vi "test2.vi"() -> ()   [LabVIEW 2012]
uses:
  G_SEN.vi
panel:
  out "n0":i32
  out "errorsum":dbl[](array[numeric])
  out "seed0":bool[](array[boolean])
  out "y":dbl[](array[numeric])
  out "x":dbl[](array[numeric])
  out "Array 4":dbl[][](array[numeric])
  out "obs":dbl[][](array[numeric])
  out "x*y":dbl[](array[numeric])
  out "Array":dbl[][](array[numeric])
  out "XY Graph 2":cluster{"Y":dbl[], "Y":dbl[]}[](graph)
  out "Array 3":dbl[](array[numeric])
  out "Array 2":cluster{dbl[][]}[](array[cluster])
  out "error out":errorcluster
  out "XY Graph":cluster{"Y":dbl[], "Y":dbl[]}[](graph)
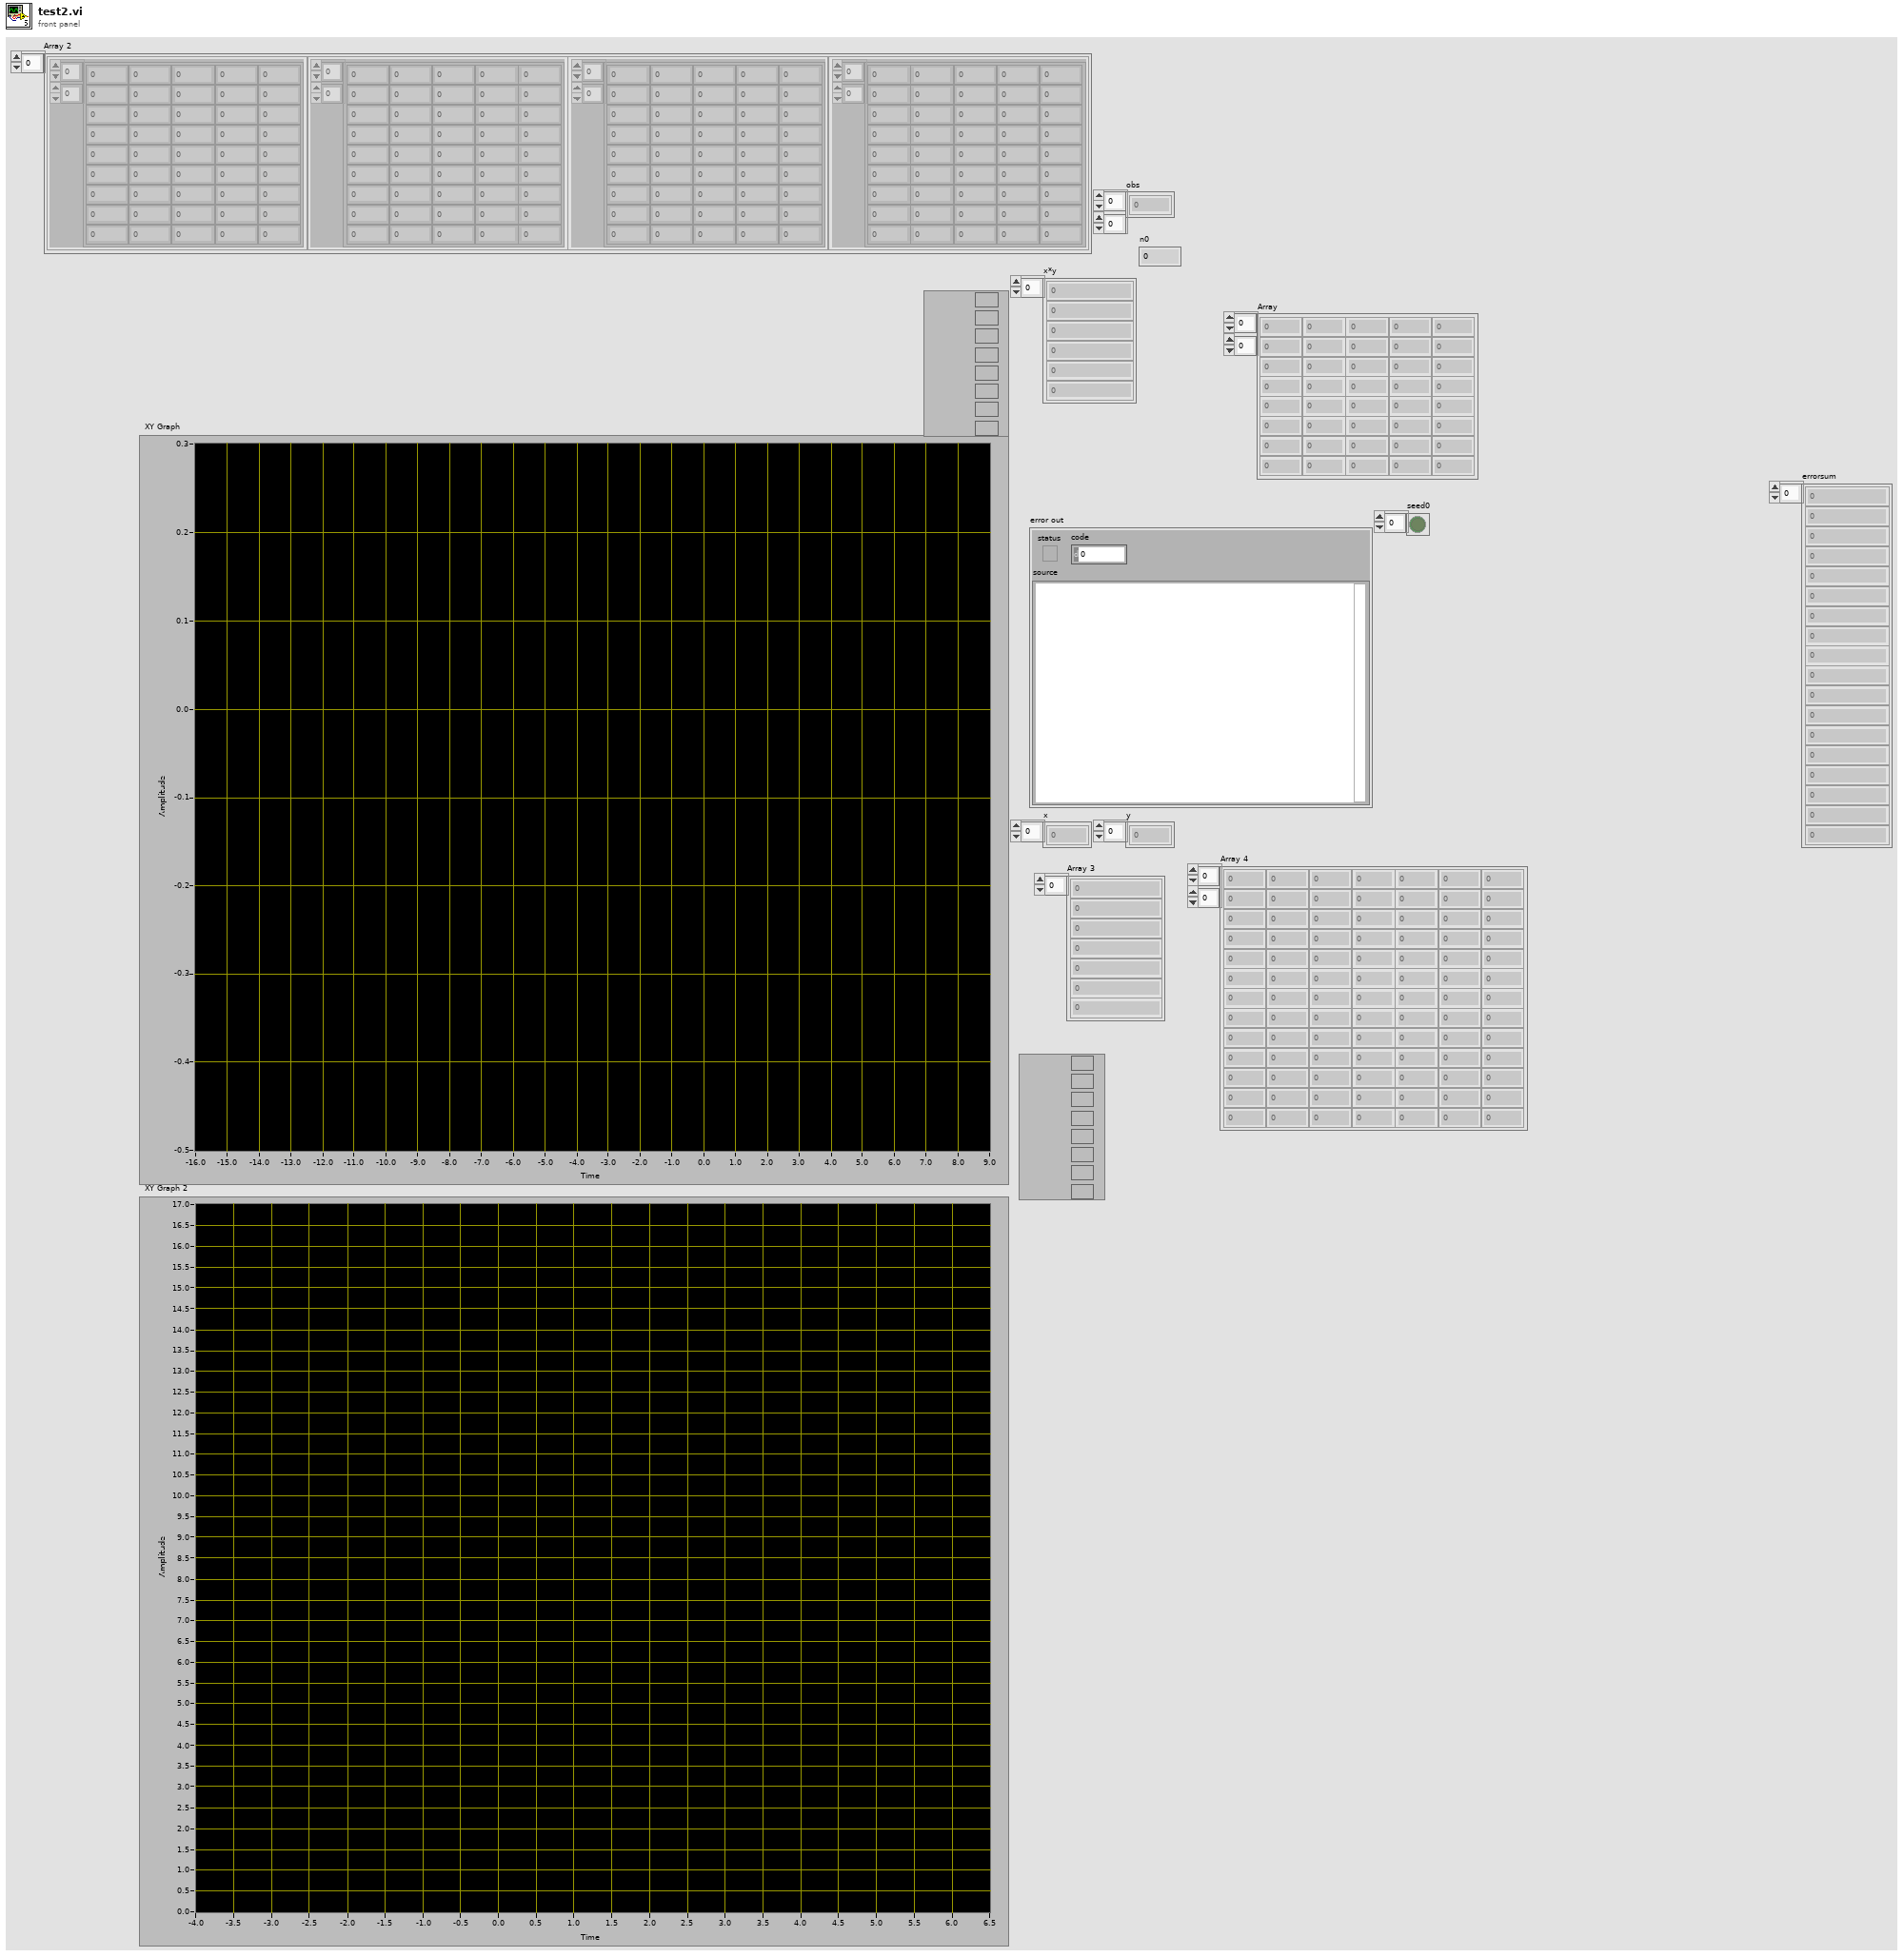
[diagram p1: front panel]
types:
  T1 = cluster{i16, "element":dbl, "element":dbl, "element":dbl, "element":dbl}[]
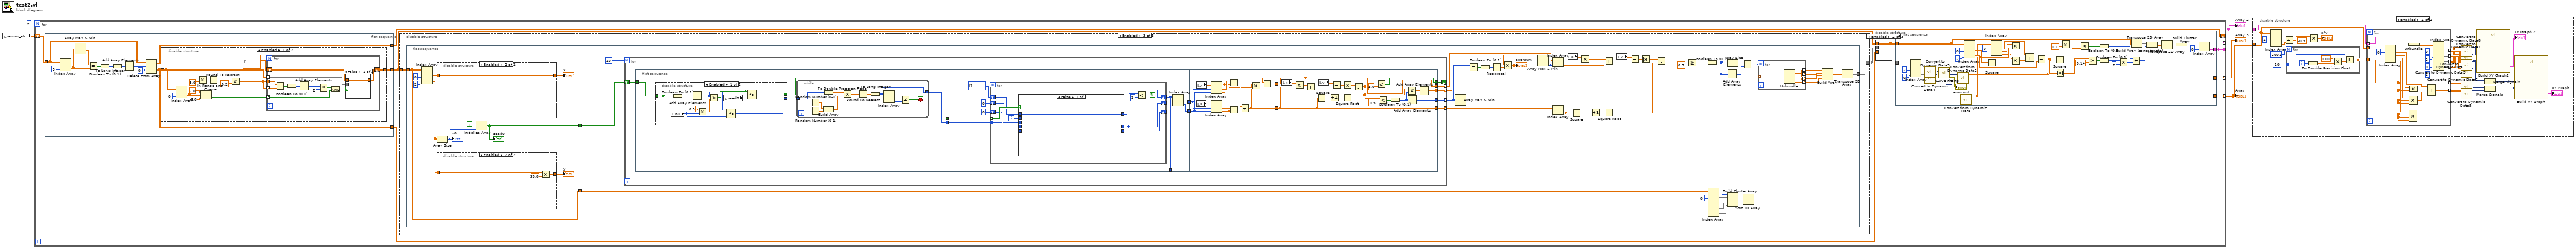
[diagram p0: block diagram]
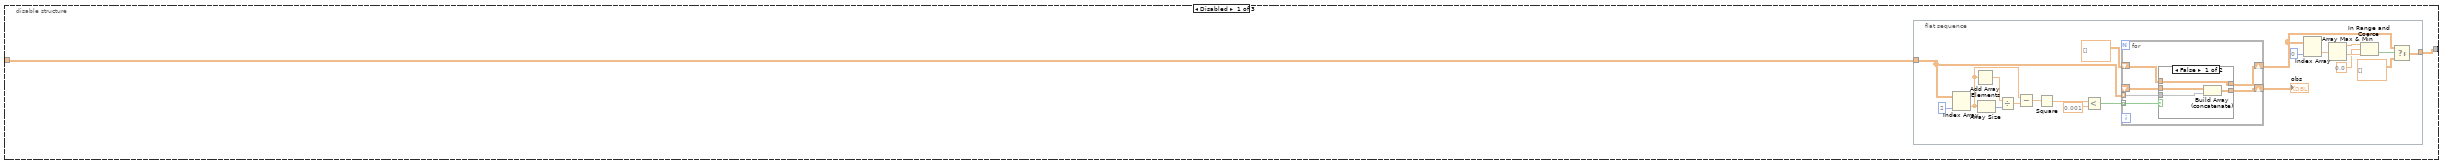
[diagram p3: hidden frame]
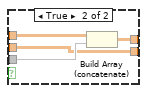
[diagram p4: hidden frame]
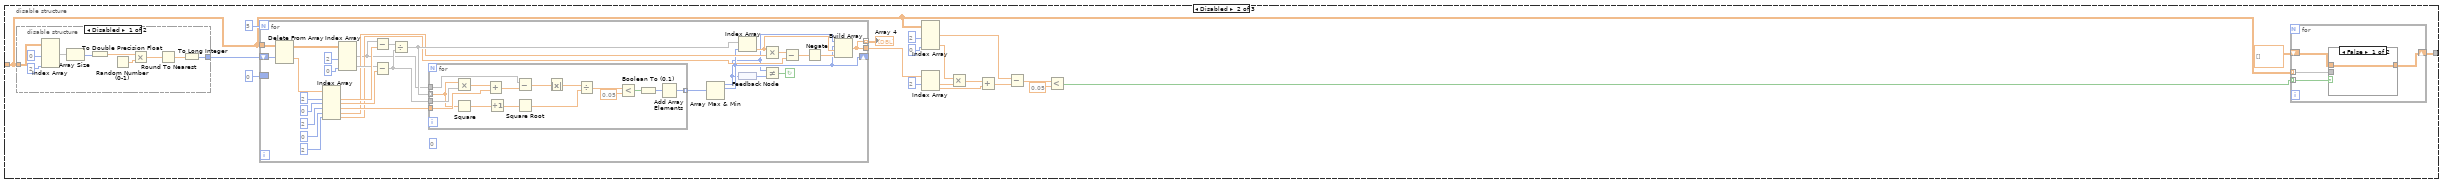
[diagram p5: hidden frame]
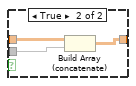
[diagram p6: hidden frame]
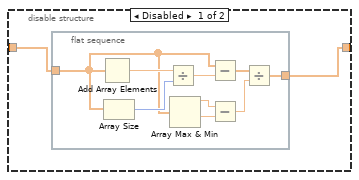
[diagram p8: hidden frame]
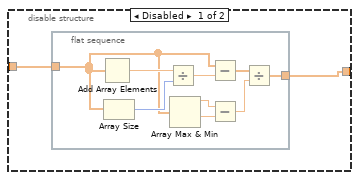
[diagram p9: hidden frame]
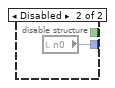
[diagram p10: hidden frame]
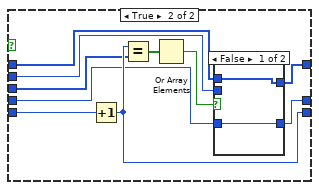
[diagram p11: hidden frame]
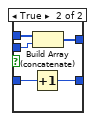
[diagram p12: hidden frame]
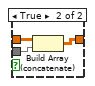
[diagram p13: hidden frame]
diagram:
  n1 = global read "G_SEN.vi" "sensor_etc"() -> (w4:dbl[][])
  n2 = for {
    N: 2 -> [_]
    shift-right: [w13] -> _
    shift-left: w4 -> [w14]
    tunnel: [w10] -> _
    tunnel: [w10] -> w2 mode=indexing
    tunnel: [w9] -> w3 mode=indexing
    tunnel: [w8] -> w1 mode=indexing
    n3 = flat-sequence {
      tunnel: w14 -> [w385]
      tunnel: [w382] -> w13
      tunnel: [w381] -> w12
      tunnel: [w380] -> w7
      frame #0 {
        n4 = Index Array(array=w385, index (col)=3 ("disabled index (col)")) -> (element=w389:dbl[])  [unwired: 1 in]
        n5 = Array Max & Min(array=w389) -> (min value=w390:dbl)  [unwired: 3 out]
        n6 = Equal?(x=w390, y=w389) -> (x = y?=w388:bool[])
        n7 = Boolean To (0,1)(Boolean=w388) -> (0, 1=w387:i16[])
        n8 = To Long Integer(number=w387) -> (32bit integer=w386:i32[])
        n9 = Add Array Elements(numeric array=w386) -> (sum=w384:i32)
        n10 = Delete From Array(array=w385, length=w384, index (row)=0) -> (deleted portion=w381:dbl[][], array with subset deleted=w382:dbl[][])  [unwired: 1 in]
        n11 = disable-structure shown="Enabled" {
          disable-tunnel: w381 -> [w397 w421]
          disable-tunnel: [w396 w421] -> w380
          frame Enabled {
            n12 = Index Array(array=w397, index (col)=0 ("disabled index (col)")) -> (element=w395:dbl[])  [unwired: 1 in]
            n13 = Multiply(x=w395, y=5.0) -> (x*y=w402:dbl[])
            n14 = In Range and Coerce(upper limit=7.0, x=w395, lower limit=-6.0) -> (In Range?=w393:bool[])  [unwired: 1 out]
            n15 = Round To Nearest(number=w402) -> (nearest integer value=w401:dbl[])
            n16 = Multiply(x=w401, y=0.2) -> (x*y=w399:dbl[])
            n17 = for {
              tunnel: w399 -> [w409] mode=indexing
              tunnel: w399 -> [w416]
              shift-right: [w412] -> w396
              shift-left: dbl[][] [] -> [w413]
              tunnel: w397 -> [w414] mode=indexing
              tunnel: w393 -> [w408] mode=indexing
              n18 = Equal?(x=w416, y=w409) -> (x = y?=w405:bool[])
              n19 = Boolean To (0,1)(Boolean=w405) -> (0, 1=w415:i16[])
              n20 = Add Array Elements(numeric array=w415) -> (sum=w411:i16)
              n21 = Less Or Equal?(x=w411, y=i16 2) -> (x <= y?=w407:bool)
              n22 = And(x=w407, y=w408) -> (x .and. y?=w406:bool)
              n23 = case shown="False" w406 {
                tunnel: w414 -> [_ w420]
                tunnel: w413 -> [w417 w419]
                tunnel: [w417 w418] -> w412
                frame False {
                }
                frame True {
                  n24 = Build Array (concatenate)(w419, w420) -> (w418:dbl[][])
                }
              }
            }
          }
          frame Disabled {
          }
        }
      }
    }
    n25 = disable-structure shown="Enabled" {
      disable-tunnel: [w16 w54 w137] -> w11
      disable-tunnel: w7 -> [w15 w56 w138]
      frame Disabled {
        n26 = flat-sequence {
          tunnel: [w37] -> w16
          tunnel: w15 -> [w36]
          frame #0 {
            n27 = Index Array(array=w36, index (col)=2 ("disabled index (col)")) -> (element=w23:dbl[])  [unwired: 1 in]
            n28 = Add Array Elements(numeric array=w23) -> (sum=w26:dbl)
            n29 = Array Size(array=w23) -> (size(s)=w22:i32)
            n30 = Divide(x=w26, y=w22) -> (x/y=w25:dbl)
            n31 = Subtract(x=w23, y=w25) -> (x-y=w24:dbl[])
            n32 = Square(x=w24) -> (x^2=w21:dbl[])
            n33 = Less?(x=w21, y=0.001) -> (x < y?=w19:bool[])
            n34 = for {
              tunnel: w36 -> [w42] mode=indexing
              tunnel: w19 -> [w43] mode=indexing
              shift-right: [w40] -> w29
              shift-left: dbl[][] [] -> [w41]
              shift-right: [w38] -> w17
              shift-left: _ -> [w39]
              n35 = case shown="False" w43 {
                tunnel: w42 -> [w46 w51]
                tunnel: w41 -> [w47 w50]
                tunnel: [w47 w49] -> w40
                tunnel: w39 -> [w45 w48]
                tunnel: [w44 w48] -> w38
                frame False {
                  n36 = Build Array (concatenate)(w45, w46) -> (w44:dbl[][])
                }
                frame True {
                  n37 = Build Array (concatenate)(w50, w51) -> (w49:dbl[][])
                }
              }
            }
            "obs" <- w17
            n38 = Index Array(array=w29, index (col)=0 ("disabled index (col)")) -> (element=w34:dbl[])  [unwired: 1 in]
            n39 = Array Max & Min(array=w34) -> (max value=w33:dbl, min value=w32:dbl)  [unwired: 2 out]
            n40 = In Range and Coerce(upper limit=w33, x=0.0, lower limit=w32) -> (In Range?=w30:bool)  [unwired: 1 out]
            n41 = Select(t=w29, s=w30, f=dbl[][] []) -> (s? t:f=w37:dbl[][])
          }
        }
      }
      frame Disabled {
        n42 = disable-structure shown="Disabled" {
          disable-tunnel: w56 -> [w85 _]
          disable-tunnel: [w80 _] -> w71
          frame Disabled {
            n43 = Index Array(array=w85, index (col) #1=0 ("disabled index (col)"), index (col) #2=2 ("index (col)")) -> (element #1=w87:dbl[])  [unwired: 2 in, 1 out]
            n44 = Array Size(array=w87) -> (size(s)=w86:i32)
            n45 = To Double Precision Float(number=w86) -> (double precision float=w84:dbl)
            n46 = Random Number (0-1)() -> (number: 0 to 1=w83:dbl)
            n47 = Multiply(x=w84, y=w83) -> (x*y=w82:dbl)
            n48 = Round To Nearest(number=w82) -> (nearest integer value=w81:dbl)
            n49 = To Long Integer(number=w81) -> (32bit integer=w80:i32)
          }
          frame Enabled {
          }
        }
        n50 = for {
          N: 5 -> [_]
          tunnel: w56 -> [w120]
          tunnel: [w90] -> w67
          shift-right: [w94] -> _
          shift-left: w71 -> [w119]
          tunnel: [w90] -> w53 mode=indexing
          border: i16 0 -> [_]
          stop <- w91 continue-if-true
          (unwired) i16 0
          n51 = Delete From Array(array=w120, index (row)=w119) -> (deleted portion=w115:dbl[], array with subset deleted=w118:dbl[][])  [unwired: 2 in]
          n52 = Index Array(array=w115, index #1=2 ("disabled index (col)"), index #2=0 ("index (col)"), index #3=2 ("index"), index #4=0 ("index"), index #5=2 ("index")) -> (element #1=w112:dbl, element #2=w110:dbl, element #3=w106:dbl, element #4=w102:dbl, element #5=w99:dbl)
          n53 = Index Array(array=w118, index (col) #1=2 ("disabled index (col)"), index (col) #2=0 ("index (col)")) -> (element #1=w95:dbl[], element #2=w111:dbl[])  [unwired: 2 in]
          n54 = Subtract(x=w95, y=w112) -> (x-y=w109:dbl[])
          n55 = Subtract(x=w111, y=w110) -> (x-y=w108:dbl[])
          n56 = Divide(x=w109, y=w108) -> (x/y=w104:dbl[])
          n57 = for {
            tunnel: w104 -> [w128] mode=indexing
            tunnel: w108 -> [w136]
            tunnel: w106 -> [w134]
            tunnel: w95 -> [w132]
            tunnel: [w121] -> w105 mode=indexing
            n58 = Multiply(x=w128, y=w136) -> (x*y=w135:dbl[])
            n59 = Square(x=w128) -> (x^2=w127:dbl)
            n60 = Add(x=w135, y=w134) -> (x+y=w133:dbl[])
            n61 = Increment(x=w127) -> (x+1=w126:dbl)
            n62 = Subtract(x=w132, y=w133) -> (x-y=w131:dbl[])
            n63 = Square Root(x=w126) -> (sqrt(x)=w125:dbl)
            n64 = Absolute Value(x=w131) -> (abs(x)=w124:dbl[])
            n65 = Divide(x=w124, y=w125) -> (x/y=w123:dbl[])
            n66 = Less?(x=w123, y=0.05) -> (x < y?=w129:bool[])
            n67 = Boolean To (0,1)(Boolean=w129) -> (0, 1=w122:i16[])
            n68 = Add Array Elements(numeric array=w122) -> (sum=w121:i16)
          }
          n69 = Array Max & Min(array=w105) -> (max value=w92:i16, max index (indices)=w94:i32)  [unwired: 2 out]
          n70 = Index Array(array=w104, index=w94) -> (element=w96:dbl)
          n71 = feedback-in #1(w92) -> ()
          n72 = feedback #1() -> (w93:i16)
          n73 = Multiply(x=w96, y=w102) -> (x*y=w101:dbl)
          n74 = Not Equal?(x=w92, y=w93) -> (x != y?=w91:bool)
          n75 = Subtract(x=w101, y=w99) -> (x-y=w98:dbl)
          n76 = Negate(x=w98) -> (-x=w97:dbl)
          n77 = Build Array(w92, w94, w96, w97) -> (w90:dbl[])
        }
        "Array 4" <- w53
        n78 = Index Array(array=w56, index (col) #1=2 ("disabled index (col)"), index (col) #2=0 ("index (col)")) -> (element #1=w60:dbl[], element #2=w64:dbl[])  [unwired: 2 in]
        n79 = Index Array(array=w67, index #1=2 ("index")) -> (element #1=w65:dbl, element #2=w62:dbl)  [unwired: 1 in]
        n80 = Multiply(x=w64, y=w65) -> (x*y=w63:dbl[])
        n81 = Add(x=w63, y=w62) -> (x+y=w61:dbl[])
        n82 = Subtract(x=w60, y=w61) -> (x-y=w58:dbl[])
        n83 = Less?(x=w58, y=0.05) -> (x < y?=w57:bool[])
        n84 = for {
          tunnel: w57 -> [w75] mode=indexing
          tunnel: w56 -> [w74] mode=indexing
          shift-right: [w73] -> w54
          shift-left: dbl[][] [] -> [w72]
          n85 = case shown="False" w75 {
            tunnel: w74 -> [_ w79]
            tunnel: [w76 w78] -> w73
            tunnel: w72 -> [w76 w77]
            frame False {
            }
            frame True {
              n86 = Build Array (concatenate)(w77, w79) -> (w78:dbl[][])
            }
          }
        }
      }
      frame Enabled {
        n87 = flat-sequence {
          tunnel: w138 -> [w145]
          tunnel: [w146] -> w140
          tunnel: [w145] -> w139
          tunnel: w140 -> [w220]
          tunnel: w139 -> [w205]
          tunnel: [w194] -> w137
          frame #0 {
            n88 = Index Array(array=w145, index (col) #1=0 ("disabled index (col)"), index (col) #2=2 ("index (col)")) -> (element #1=w144:dbl[], element #2=w142:dbl[])  [unwired: 2 in]
            n89 = disable-structure shown="Enabled" {
              disable-tunnel: w144 -> [w152 w162]
              disable-tunnel: [w151 w162] -> w143
              frame Disabled {
                n90 = flat-sequence {
                  tunnel: w152 -> [w156]
                  tunnel: [w153] -> w151
                  frame #0 {
                    n91 = Add Array Elements(numeric array=w156) -> (sum=w159:dbl)
                    n92 = Array Size(array=w156) -> (size(s)=w158:i32)
                    n93 = Divide(x=w159, y=w158) -> (x/y=w157:dbl)
                    n94 = Array Max & Min(array=w156) -> (max value=w161:dbl, min value=w160:dbl)  [unwired: 2 out]
                    n95 = Subtract(x=w156, y=w157) -> (x-y=w155:dbl[])
                    n96 = Subtract(x=w161, y=w160) -> (x-y=w154:dbl)
                    n97 = Divide(x=w155, y=w154) -> (x/y=w153:dbl[])
                  }
                }
              }
              frame Enabled {
              }
            }
            "x" <- w143
            n98 = Array Size(array=w142) -> (size(s)=w148:i32)
            "n0" <- w148
            n99 = disable-structure shown="Enabled" {
              disable-tunnel: w142 -> [w164 w176]
              disable-tunnel: [w163 w175] -> w141
              frame Disabled {
                n100 = flat-sequence {
                  tunnel: w164 -> [w168]
                  tunnel: [w165] -> w163
                  frame #0 {
                    n101 = Add Array Elements(numeric array=w168) -> (sum=w171:dbl)
                    n102 = Array Size(array=w168) -> (size(s)=w170:i32)
                    n103 = Divide(x=w171, y=w170) -> (x/y=w169:dbl)
                    n104 = Array Max & Min(array=w168) -> (max value=w173:dbl, min value=w172:dbl)  [unwired: 2 out]
                    n105 = Subtract(x=w168, y=w169) -> (x-y=w167:dbl[])
                    n106 = Subtract(x=w173, y=w172) -> (x-y=w166:dbl)
                    n107 = Divide(x=w167, y=w166) -> (x/y=w165:dbl[])
                  }
                }
              }
              frame Enabled {
                n108 = Multiply(x=w176, y=30.0) -> (x*y=w175:dbl[])
              }
            }
            "y" <- w141
            n109 = Initialize Array(TRUE, w148) -> (w146:bool[])
            "seed0" <- w146
          }
          frame #1 {
            n110 = for {
              N: 20 -> [_]
              shift-right: [w232] -> _
              shift-left: w220 -> [w235]
              tunnel: [w231] -> w218 mode=indexing
              tunnel: [w230] -> w217 mode=indexing
              tunnel: [w227] -> w184 mode=indexing
              tunnel: [w226] -> w188 mode=indexing
              n111 = flat-sequence {
                tunnel: w235 -> [w241]
                tunnel: [w238] -> w234
                tunnel: [w240] -> w233
                tunnel: [w266] -> w237
                tunnel: [w265] -> w236
                tunnel: w234 -> [w271]
                tunnel: w233 -> [w269]
                tunnel: [w264] -> _
                tunnel: w237 -> [w313]
                tunnel: w236 -> [w312]
                tunnel: [w304] -> w229
                tunnel: [w303] -> w228
                tunnel: [w330] -> w232
                tunnel: [w321] -> w231
                tunnel: [w329] -> w230
                tunnel: w229 -> [w329]
                tunnel: w228 -> [w321]
                tunnel: [w325] -> w227
                tunnel: [w324] -> w226
                frame #0 {
                  n112 = disable-structure shown="Enabled" {
                    disable-tunnel: w241 -> [w245 _]
                    disable-tunnel: [w247 w252] -> w239
                    disable-tunnel: [w244 _] -> w238
                    frame Enabled {
                      n113 = local read "n0"() -> (w246:i32)
                      n114 = Boolean To (0,1)(Boolean=w245) -> (0, 1=w251:i16[])
                      n115 = Add Array Elements(numeric array=w251) -> (sum=w248:i16)
                      n116 = Multiply(x=0.5, y=w246) -> (x*y=w249:dbl)
                      n117 = Greater?(x=w248, y=w249) -> (0:w242:bool)
                      n118 = local read "seed0"() -> (w243:bool[])
                      n119 = Select(t=w248, s=w242, f=w246) -> (s? t:f=w247:i32)
                      n120 = Select(t=w245, s=w242, f=w243) -> (s? t:f=w244:bool[])
                    }
                    frame Disabled {
                      n121 = local read "n0"() -> (w252:i32)
                    }
                  }
                  n122 = while {
                    tunnel: w239 -> [w254]
                    tunnel: [w253] -> w240
                    stop <- w255 stop-if-true
                    n123 = Random Number (0-1)() -> (number: 0 to 1=w263:dbl)
                    n124 = Random Number (0-1)() -> (number: 0 to 1=w262:dbl)
                    n125 = Build Array(w263, w262) -> (w261:dbl[])
                    n126 = To Double Precision Float(number=w254) -> (double precision float=w258:dbl)
                    n127 = Multiply(x=w258, y=w261) -> (x*y=w260:dbl[])
                    n128 = Round To Nearest(number=w260) -> (nearest integer value=w259:dbl[])
                    n129 = To Long Integer(number=w259) -> (32bit integer=w253:i32[])
                    n130 = Index Array(array=w253) -> (element #1=w257:i32, element #2=w256:i32)  [unwired: 2 in]
                    n131 = Not Equal?(x=w257, y=w256) -> (x != y?=w255:bool)
                  }
                }
                frame #1 {
                  n132 = for {
                    tunnel: w271 -> [w282] mode=indexing
                    shift-right: [w280] -> _
                    shift-left: 0 -> [w281]
                    tunnel: w269 -> [w279]
                    shift-right: [w277] -> w264
                    shift-left: i32[] [] -> [w276]
                    shift-right: [w274] -> _
                    shift-left: 0 -> [w275]
                    i -> [w278]
                    stop <- w272 continue-if-true
                    n133 = case shown="False" w282 {
                      tunnel: w281 -> [w285 w295]
                      tunnel: [w285 w294] -> w280
                      tunnel: w279 -> [_ w293]
                      tunnel: w278 -> [_ w290]
                      tunnel: [w284 w289] -> w277
                      tunnel: w276 -> [w284 w288]
                      tunnel: w275 -> [w283 w287]
                      tunnel: [w283 w286] -> w274
                      frame False {
                      }
                      frame True {
                        n134 = Increment(x=w295) -> (x+1=w294:i32)
                        n135 = Equal?(x=w294, y=w293) -> (x = y?=w292:bool[])
                        n136 = Or Array Elements(Boolean array=w292) -> (logical OR=w291:bool)
                        n137 = case shown="False" w291 {
                          tunnel: w290 -> [_ w302]
                          tunnel: [w297 w301] -> w289
                          tunnel: w288 -> [w297 w300]
                          tunnel: w287 -> [w296 w299]
                          tunnel: [w296 w298] -> w286
                          frame False {
                          }
                          frame True {
                            n138 = Increment(x=w299) -> (x+1=w298:i32)
                            n139 = Build Array (concatenate)(w300, w302) -> (w301:i32[])
                          }
                        }
                      }
                    }
                    n140 = Less?(x=w274, y=2) -> (x < y?=w272:bool)
                  }
                  n141 = Index Array(array=w264) -> (element #1=w266:i32, element #2=w265:i32)  [unwired: 2 in]
                }
                frame #2 {
                  n142 = local read "y"() -> (w314:dbl[])
                  n143 = local read "x"() -> (w315:dbl[])
                  n144 = Index Array(array=w315, index #1=w313, index #2=w312) -> (element #1=w309:dbl, element #2=w306:dbl)
                  n145 = Index Array(array=w314, index #1=w313, index #2=w312) -> (element #1=w307:dbl, element #2=w305:dbl)
                  n146 = Subtract(x=w307, y=w305) -> (x-y=w311:dbl)
                  n147 = Subtract(x=w309, y=w306) -> (x-y=w310:dbl)
                  n148 = Divide(x=w311, y=w310) -> (x/y=w303:dbl)
                  n149 = Multiply(x=w303, y=w306) -> (x*y=w308:dbl)
                  n150 = Subtract(x=w305, y=w308) -> (x-y=w304:dbl)
                }
                frame #3 {
                  n151 = local read "x"() -> (w328:dbl[])
                  n152 = Multiply(x=w328, y=w321) -> (x*y=w335:dbl[])
                  n153 = Add(x=w335, y=w329) -> (x+y=w334:dbl[])
                  n154 = Square(x=w321) -> (x^2=w320:dbl)
                  n155 = local read "y"() -> (w333:dbl[])
                  n156 = Increment(x=w320) -> (x+1=w319:dbl)
                  n157 = Subtract(x=w333, y=w334) -> (x-y=w332:dbl[])
                  n158 = Absolute Value(x=w332) -> (abs(x)=w318:dbl[])
                  n159 = Square Root(x=w319) -> (sqrt(x)=w317:dbl)
                  n160 = Divide(x=w318, y=w317) -> (x/y=w316:dbl[])
                  n161 = Less?(x=w316, y=3.0) -> (x < y?=w330:bool[])
                  n162 = Less?(x=w316, y=0.5) -> (x < y?=w322:bool[])
                  n163 = Boolean To (0,1)(Boolean=w322) -> (0, 1=w326:i16[])
                  n164 = Multiply(x=w316, y=w326) -> (x*y=w327:dbl[])
                  n165 = Add Array Elements(numeric array=w326) -> (sum=w324:i16)
                  n166 = Add Array Elements(numeric array=w327) -> (sum=w325:dbl)
                }
              }
            }
            n167 = Array Max & Min(array=w188) -> (max value=w189:i16)  [unwired: 3 out]
            n168 = Equal?(x=w188, y=w189) -> (x = y?=w187:bool[])
            n169 = Boolean To (0,1)(Boolean=w187) -> (0, 1=w186:i16[])
            n170 = Reciprocal(x=w186) -> (1/x=w185:dbl[])
            n171 = Multiply(x=w184, y=w185) -> (x*y=w183:dbl[])
            "errorsum" <- w183
            n172 = Array Max & Min(array=w183) -> (min index (indices)=w216:i32)  [unwired: 3 out]
            n173 = Index Array(array=w217, index=w216) -> (element=w209:dbl)
            n174 = Index Array(array=w218, index=w216) -> (element=w179:dbl)
            n175 = local read "x"() -> (w215:dbl[])
            n176 = Square(x=w179) -> (x^2=w180:dbl)
            n177 = Multiply(x=w215, y=w179) -> (x*y=w210:dbl[])
            n178 = Increment(x=w180) -> (x+1=w181:dbl)
            n179 = Add(x=w210, y=w209) -> (x+y=w211:dbl[])
            n180 = Square Root(x=w181) -> (sqrt(x)=w182:dbl)
            n181 = local read "y"() -> (w212:dbl[])
            n182 = Subtract(x=w212, y=w211) -> (x-y=w213:dbl[])
            n183 = Absolute Value(x=w213) -> (abs(x)=w178:dbl[])
            n184 = Divide(x=w178, y=w182) -> (x/y=w177:dbl[])
            n185 = Greater Or Equal?(x=w177, y=0.5) -> (x >= y?=w208:bool[])
            n186 = Boolean To (0,1)(Boolean=w208) -> (0, 1=w193:i16[])
            n187 = Index Array(array=w205, index (col) #1=0 ("disabled index (col)")) -> (element #1=w203:dbl[], element #2=w202:dbl[], element #3=w201:dbl[], element #4=w200:dbl[])  [unwired: 7 in]
            n188 = Add Array Elements(numeric array=w193) -> (sum=w191:i16)
            n189 = Array Size(array=w193) -> (size(s)=w192:i32)
            n190 = Build Cluster Array(w193, w203, w202, w201, w200) -> (w207:T1)
            n191 = Subtract(x=w192, y=w191) -> (x-y=w190:i32)
            n192 = Sort 1D Array(array=w207) -> (sorted array=w206:T1)
            n193 = for {
              N: w190 -> [_]
              tunnel: w206 -> [w225] mode=indexing
              tunnel: [w224] -> w199 mode=indexing
              tunnel: [w223] -> w198 mode=indexing
              tunnel: [w222] -> w197 mode=indexing
              tunnel: [w221] -> w196 mode=indexing
              n194 = Unbundle(w225) -> ("element"=w224:dbl, "element"=w223:dbl, "element"=w222:dbl, "element"=w221:dbl)  [unwired: 1 out]
            }
            n195 = Build Array(w199, w198, w197, w196) -> (w195:dbl[][])
            n196 = Transpose 2D Array(2D array=w195) -> (transposed array=w194:dbl[][])
          }
        }
      }
    }
    n197 = disable-structure shown="Enabled" {
      disable-tunnel: w12 -> [w422 _ _]
      disable-tunnel: [w422 w423 w424] -> w6
      disable-tunnel: w11 -> [_ _ w424]
      disable-tunnel: w7 -> [_ w423 _]
      frame Disabled {
      }
      frame Enabled {
      }
      frame Disabled {
      }
    }
    n198 = flat-sequence {
      tunnel: w11 -> [w340]
      tunnel: [w339] -> w10
      tunnel: [w338] -> w9
      tunnel: [w337] -> w8
      tunnel: w6 -> [w336]
      frame #0 {
        n199 = Index Array(array=w340, index (col) #1=2 ("disabled index (col)"), index (col) #2=0 ("index (col)")) -> (element #1=w370:dbl[], element #2=w374:dbl[])  [unwired: 2 in]
        n200 = call "Convert to Dynamic Data3"("Array"=w370) -> ("Dynamic Data Type"=w375:dynamicdata)  [unwired: 3 in]
        n201 = call "Convert to Dynamic Data4"("Array"=w374) -> ("Dynamic Data Type"=w373:dynamicdata)  [unwired: 3 in]
        n202 = call "Curve Fitting"("Locations"=w373, "Signals"=w375) -> ("error out"=→"error out":errorcluster, "mean squared error"=w371:dynamicdata, "polynomial coefficients"=w372:dynamicdata)  [unwired: 5 in, 2 out]
        n203 = call "Convert from Dynamic Data2"("Dynamic Data Type"=w371) -> ("Scalar"=w338:dbl)  [unwired: 3 in]
        n204 = call "Convert from Dynamic Data"("Dynamic Data Type"=w372) -> ("Array"=w337:dbl[])  [unwired: 3 in]
        n205 = Index Array(array=w336, index (col) #1=0 ("disabled index (col)"), index (col) #2=2 ("index (col)")) -> (element #1=w366:dbl[], element #2=w358:dbl[])  [unwired: 2 in]
        n206 = Square(x=w366) -> (x^2=w364:dbl[])
        n207 = Index Array(array=w337, index #1=0 ("index")) -> (element #1=w363:dbl, element #2=w367:dbl, element #3=w365:dbl)  [unwired: 2 in]
        n208 = Multiply(x=w367, y=w366) -> (x*y=w362:dbl[])
        n209 = Multiply(x=w365, y=w364) -> (x*y=w361:dbl[])
        n210 = Compound Arithmetic op=ADD(w363, w362, w361) -> (w359:dbl[])
        n211 = Subtract(x=w359, y=w358) -> (x-y=w350:dbl[])
        n212 = Square(x=w350) -> (x^2=w355:dbl[])
        n213 = Absolute Value(x=w350) -> (abs(x)=w349:dbl[])
        n214 = Multiply(x=w338, y=1.1) -> (x*y=w356:dbl)
        n215 = Less?(x=w356, y=w355) -> (x < y?=w353:bool[])
        n216 = Greater?(x=w349, y=0.14) -> (0:w347:bool[])
        n217 = Boolean To (0,1)(Boolean=w353) -> (0, 1=w346:i16[])
        n218 = Boolean To (0,1)(Boolean=w347) -> (0, 1=w344:i16[])
        n219 = Multiply(x=w344, y=i16 2) -> (x*y=w342:i16[])
        n220 = Add(x=w346, y=w342) -> (x+y=w345:i16[])
        n221 = Transpose 2D Array(2D array=w336) -> (transposed array=w354:dbl[][])
        n222 = Build Array (concatenate)(w354, w345) -> (w352:dbl[][])
        n223 = Transpose 2D Array(2D array=w352) -> (transposed array=w351:dbl[][])
        n224 = Build Cluster Array(w351) -> (w379:cluster{dbl[][]}[])
        n225 = Index Array(array=w379, index=0) -> (element=w339:cluster{dbl[][]})
      }
    }
  }
  "Array 2" <- w2
  "Array 3" <- w3
  "Array" <- w1
  n226 = disable-structure shown="Enabled" {
    disable-tunnel: w2 -> [w438 _]
    disable-tunnel: w1 -> [w431 _]
    frame Enabled {
      n227 = Index Array(array=w431, index (col) #1=1 ("disabled index (col)")) -> (element #1=w429:dbl[], element #2=w428:dbl[])  [unwired: 3 in]
      n228 = Divide(x=w429, y=w428) -> (x/y=w427:dbl[])
      n229 = for {
        N: 2001 -> [_]
        tunnel: -10 -> [w454]
        tunnel: [w452] -> w448 mode=indexing
        i -> [w457]
        n230 = To Double Precision Float(number=w457) -> (double precision float=w456:dbl)
        n231 = Multiply(x=0.01, y=w456) -> (x*y=w453:dbl)
        n232 = Add(x=w454, y=w453) -> (x+y=w452:dbl)
      }
      n233 = Multiply(x=w427, y=-0.5) -> (x*y=→"x*y":dbl[])
      n234 = for {
        tunnel: w438 -> [w478] mode=indexing
        tunnel: [w473] -> w447 mode=indexing
        tunnel: [w472] -> w446 mode=indexing
        tunnel: w448 -> [w459]
        tunnel: w431 -> [w471] mode=indexing
        tunnel: [w459] -> w440 mode=indexing
        tunnel: [w464] -> w443 mode=indexing
        tunnel: [w462] -> w436 mode=indexing
        tunnel: [w461] -> w433 mode=indexing
        n235 = Index Array(array=w471, index #1=0 ("index")) -> (element #1=w467:dbl, element #2=w469:dbl, element #3=w468:dbl, element #4=w460:dbl)  [unwired: 3 in]
        n236 = Unbundle(w478) -> (w475:dbl[][])
        n237 = Compound Arithmetic op=MULTIPLY(w460, w459, w459, w459) -> (w458:dbl[])
        n238 = Compound Arithmetic op=MULTIPLY(w468, w459, w459) -> (w465:dbl[])
        n239 = Compound Arithmetic op=MULTIPLY(w469, w459) -> (w466:dbl[])
        n240 = Compound Arithmetic op=ADD(w467, w466, w465, w458) -> (w464:dbl[])
        n241 = Index Array(array=w475, index (col) #1=0 ("disabled index (col)"), index (col) #2=2 ("index (col)"), index (col) #3=0 ("index (col)"), index (col) #4=1 ("index (col)")) -> (element #1=w473:dbl[], element #2=w472:dbl[], element #3=w461:dbl[], element #4=w462:dbl[])  [unwired: 4 in]
      }
      n242 = call "Convert to Dynamic Data8"("2D Array"=w433) -> ("Dynamic Data Type"=w432:dynamicdata)  [unwired: 3 in]
      n243 = call "Convert to Dynamic Data7"("2D Array"=w436) -> ("Dynamic Data Type"=w435:dynamicdata)  [unwired: 3 in]
      n244 = call "Convert to Dynamic Data"("2D Array"=w447) -> ("Dynamic Data Type"=w437:dynamicdata)  [unwired: 3 in]
      n245 = call "Convert to Dynamic Data2"("2D Array"=w446) -> ("Dynamic Data Type"=w445:dynamicdata)  [unwired: 3 in]
      n246 = call "Convert to Dynamic Data6"("2D Array"=w440) -> ("Dynamic Data Type"=w439:dynamicdata)  [unwired: 3 in]
      n247 = call "Convert to Dynamic Data5"("2D Array"=w443) -> ("Dynamic Data Type"=w442:dynamicdata)  [unwired: 3 in]
      n248 = call "Build XY Graph2"("Y Input"=w435, "X Input"=w432) -> ("XY Graph"=→"XY Graph 2":cluster{"Y":dbl[], "Y":dbl[]}[])  [unwired: 3 in, 6 out]
      n249 = Merge Signals(w437, w439) -> (w441:dynamicdata)
      n250 = Merge Signals(w445, w442) -> (w444:dynamicdata)
      n251 = call "Build XY Graph"("Y Input"=w444, "X Input"=w441) -> ("XY Graph"=→"XY Graph":cluster{"Y":dbl[], "Y":dbl[]}[])  [unwired: 3 in, 6 out]
    }
    frame Disabled {
    }
  }
